vi "ROS_Topic_Read.vi"(3 "error in (no error)":errorcluster, 5 "ROS in":T1={"topic port"=0, "Node"="", "topic"="", "type"="", "node port"=0, "error "={"status"=FALSE, "code"=0, "source"=""}, "Direction"=enum."Node", "Update (ms)"=1, "FIFO size"=1}) -> (0 "error out":errorcluster, 1 "Reply":string, 2 "ROS out":T1={"topic port"=0, "Node"="", "topic"="", "type"="", "node port"=0, "error "={"status"=FALSE, "code"=0, "source"=""}, "Direction"=enum."Node", "Update (ms)"=1, "FIFO size"=1})   [LabVIEW 2014]
doc: "Waits for a non-empty message on the ROS topic or service until Timeout."
uses:
  <userlib>/ROS for LabVIEW Software/ROS/Code/SubVIs/_ROSControl.ctl
  <userlib>/ROS for LabVIEW Software/ROS/Code/SubVIs/_ROSDirection.ctl
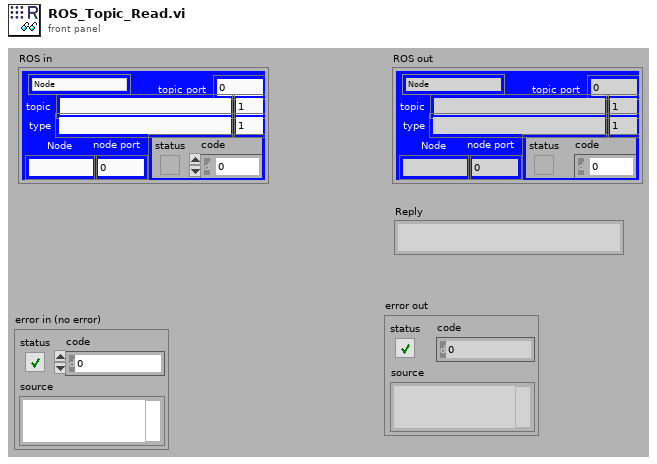
[diagram p1: front panel]
types:
  T1 = typedef "_ROSControl.ctl" = cluster{"topic port":u16, "Node":string, "topic":string, "type":string, "node port":u16, "error ":errorcluster, "Direction":T2, "Update (ms)":u16, "FIFO size":u16}
  T2 = typedef "_ROSDirection.ctl" = enum16{"Node", "Publisher", "Subscriber", "ServiceClient", "ServiceProvider"}
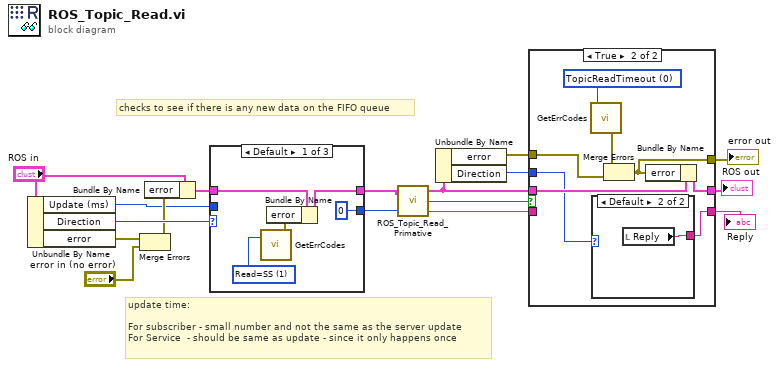
[diagram p0: block diagram]
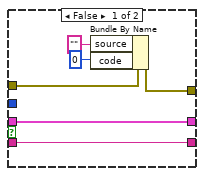
[diagram p2: hidden frame]
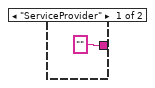
[diagram p3: hidden frame]
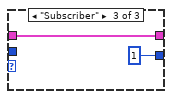
[diagram p5: hidden frame]
diagram:
  # "checks to see if there is any new data on the FIFO queue"
  # "update time:\n\nFor subscriber - small number and not the same as the server update\nFor Service  - should be same as update - since it only happens once"
  n1 = Unbundle By Name("ROS in") -> ("Update (ms)"=w1:u16, "Direction"=w17:T2, "error"=w15:errorcluster)
  n2 = Merge Errors(w15, "error in (no error)") -> (w11:errorcluster)
  n3 = Bundle By Name(cluster="ROS in", "error"=w11) -> (w12:T1)
  n4 = case shown="Default" w17 {
    tunnel: [w22 w24 w26] -> w16
    tunnel: w12 -> [w21 w24 w26]
    tunnel: [0 ("Timeout (ms)") w23 1 ("Timeout (ms)")] -> w2
    tunnel: w1 -> [_ w23 _]
    frame Default {
      w19 = u16 1 items=["TopicReadTimeout", "Read=SS", "GetQueueErr", "NoMaster", "Write=PS", "Unparse", "ServiceReply"] ("Error")
      n5 = call <userlib>:"GetErrCodes.vi"("Error"=w19) -> ("Error"=w20:errorcluster)  [unwired: 1 in]
      n6 = Bundle By Name(cluster=w21, "error"=w20) -> (w22:T1)
    }
    frame "ServiceClient", "ServiceProvider" {
    }
    frame "Subscriber" {
    }
  }
  n7 = call <userlib>:"ROS_Topic_Read_Primative.vi"("ROS in"=w16, "Timeout (ms)"=w2) -> ("ROS out"=w6:T1, "timed out?"=w10:bool, "Reply"=w8:string)
  n8 = Unbundle By Name(w6) -> ("error"=w5:errorcluster, "Direction"=w3:T2)
  n9 = case shown="True" w10 {
    tunnel: [w32 w40] -> w9
    tunnel: w8 -> [w32 _]
    tunnel: [w31 w38] -> w7
    tunnel: w6 -> [w31 w37]
    tunnel: w5 -> [w30 w39]
    tunnel: [w29 w36] -> w4
    tunnel: w3 -> [_ w35]
    frame False {
      n10 = Bundle By Name(cluster=w30, "source"="", "code"=0) -> (w29:errorcluster)
    }
    frame True {
      w34 = u16 0 items=["TopicReadTimeout", "Read=SS"] ("Error")
      n11 = call <userlib>:"GetErrCodes.vi"("Error"=w34) -> ("Error"=w33:errorcluster)  [unwired: 1 in]
      n12 = case shown="Default" w35 {
        tunnel: ["" ("Reply") w42] -> w40
        frame "ServiceProvider" {
        }
        frame Default {
          n13 = local read "Reply"() -> (w42:string)
        }
      }
      n14 = Merge Errors(w33, w39) -> (w36:errorcluster)
      n15 = Bundle By Name(cluster=w37, "error"=w36) -> (w38:T1)
    }
  }
  "ROS out" <- w7
  "error out" <- w4
  "Reply" <- w9
